vi "Insert_DI.vi"(2 "table":string, 3 "date/time string":string, 4 "error in (no error)":errorcluster, 5 "connection reference":T1, 6 "BIT (DATO)":i32=1203, 7 "Numeric (ID_SENSOR)":i32=1203) -> (0 "error out":errorcluster, 1 "connection reference out":T1)   [LabVIEW 2017]
uses:
  <vilib>/addons/database/Connection.llb/Conn ObjectReference.ctl
  <vilib>/addons/database/NI_Database_API.lvlib
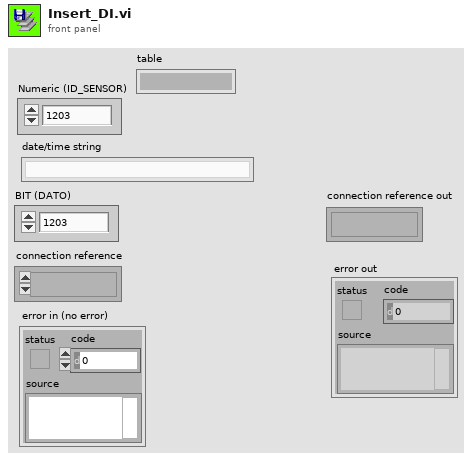
[diagram p1: front panel]
types:
  T1 = typedef "NI_Database_API.lvlib/Conn ObjectReference.ctl" = refnum<k1>
  T2 = cluster{"Numeric (ID_SENSOR)":i32, "date/time string":string, "BIT (DATO)":i32}
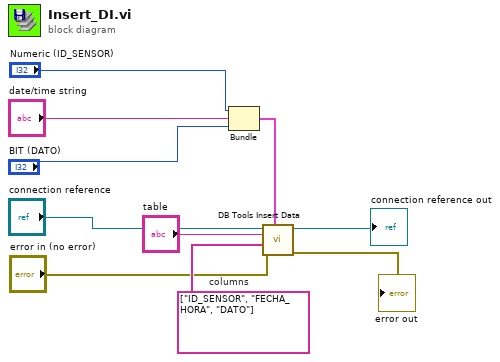
[diagram p0: block diagram]
diagram:
  w6 = string[] ["ID_SENSOR", "FECHA_HORA", "DATO"]  # columns
  n1 = Bundle("Numeric (ID_SENSOR)"="Numeric (ID_SENSOR)", "date/time string"="date/time string", "BIT (DATO)"="BIT (DATO)") -> (w9:T2)  [unwired: 1 in]
  n2 = call <vilib>:"DB Tools Insert Data.vi"("data"=w9, "error in (no error)"="error in (no error)", "columns"=w6, "table"="table", "connection reference"="connection reference") -> ("error out"=→"error out":errorcluster, "connection reference out"=→"connection reference out":T1)  [unwired: 5 in]
